vi "HIOKI PW3390 Acquisition Waveform.vi"() -> ()   [LabVIEW 2009]
doc: "Outputs the voltage and current waveforms of the specified channel."
uses:
  <instrlib>/PW3390/Common/_Initialize/HIOKI PW3390 Initialize LAN.vi
panel:
  out "error out":errorcluster
  in  "Analysis CH":enum16{"CH 1", "CH 2", "CH 3", "CH 4"}(ring)
  out "I Wave":waveform(sgl)(graph)
  out "U Wave":waveform(sgl)(graph)
  in  "IP Address":string="192.168.1.1"
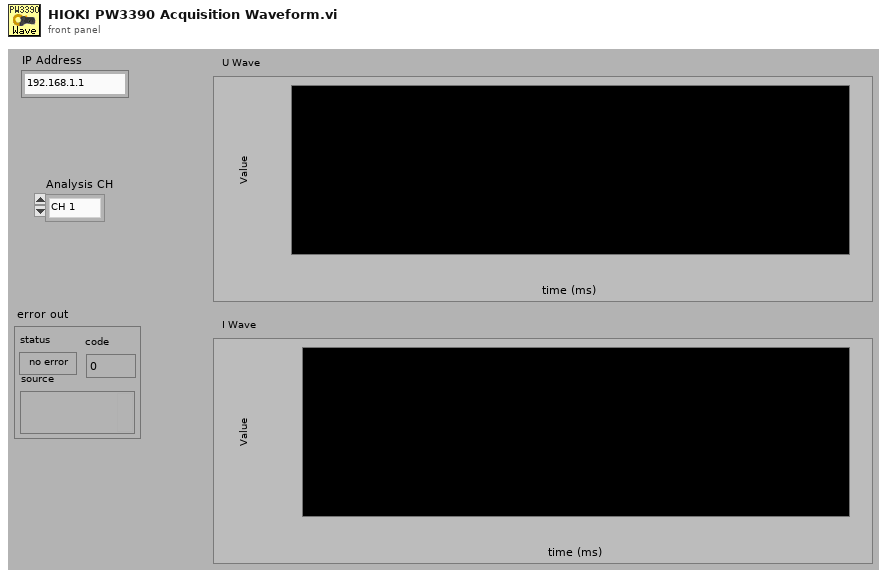
[diagram p1: front panel]
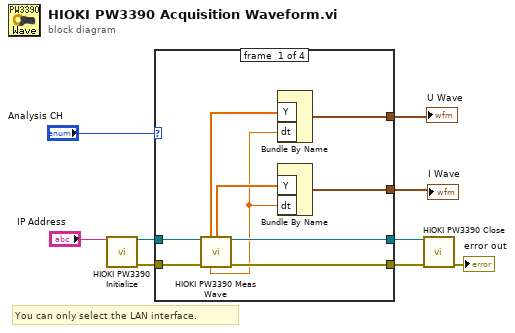
[diagram p0: block diagram]
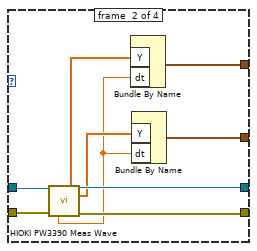
[diagram p2: hidden frame]
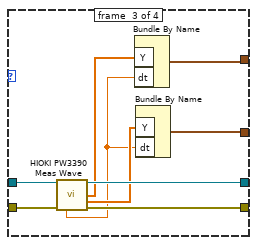
[diagram p3: hidden frame]
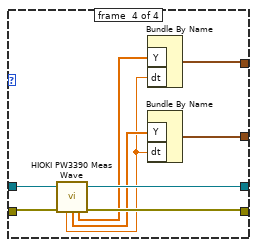
[diagram p4: hidden frame]
diagram:
  # "You can only select the LAN interface."
  n1 = call-poly <instrlib>:"HIOKI PW3390 Initialize.vi"("IP Address"="IP Address") -> ("VISA Resource out"=w5:refnum<visa-resource-name>, "error out"=w2:errorcluster)  [unwired: 12 in, 1 out]
  n2 = case shown="\"CH 1\"" "Analysis CH" {
    tunnel: [w18 w27 w36 w45] -> w7
    tunnel: [w17 w26 w35 w44] -> w6
    tunnel: w5 -> [w16 w25 w34 w43]
    tunnel: [w15 w22 w32 w40] -> w4
    tunnel: [w14 w23 w31 w41] -> w3
    tunnel: w2 -> [w13 w24 w33 w42]
    frame #0 {
      n3 = call <instrlib>:"HIOKI PW3390 Meas Wave.vi"("VISA Resource"=w16, "error in (no error)"=w13) -> ("U1 Value out"=w12:sgl[], "I1 Value out"=w11:sgl[], "VISA Resource out"=w15:refnum<visa-resource-name>, "dt out"=w10:dbl, "error out"=w14:errorcluster)  [unwired: 3 in, 6 out]
      n4 = Bundle By Name("Y"=w12, "dt"=w10) -> (w18:waveform(sgl))  [unwired: 1 in]
      n5 = Bundle By Name("Y"=w11, "dt"=w10) -> (w17:waveform(sgl))  [unwired: 1 in]
    }
    frame #1 {
      n6 = call <instrlib>:"HIOKI PW3390 Meas Wave.vi"("VISA Resource"=w25, "error in (no error)"=w24) -> ("U2 Value out"=w20:sgl[], "VISA Resource out"=w22:refnum<visa-resource-name>, "I2 Value out"=w21:sgl[], "dt out"=w19:dbl, "error out"=w23:errorcluster)  [unwired: 3 in, 6 out]
      n7 = Bundle By Name("Y"=w20, "dt"=w19) -> (w27:waveform(sgl))  [unwired: 1 in]
      n8 = Bundle By Name("Y"=w21, "dt"=w19) -> (w26:waveform(sgl))  [unwired: 1 in]
    }
    frame #2 {
      n9 = call <instrlib>:"HIOKI PW3390 Meas Wave.vi"("VISA Resource"=w34, "error in (no error)"=w33) -> ("VISA Resource out"=w32:refnum<visa-resource-name>, "U3 Value out"=w30:sgl[], "I3 Value out"=w29:sgl[], "dt out"=w28:dbl, "error out"=w31:errorcluster)  [unwired: 3 in, 6 out]
      n10 = Bundle By Name("Y"=w30, "dt"=w28) -> (w36:waveform(sgl))  [unwired: 1 in]
      n11 = Bundle By Name("Y"=w29, "dt"=w28) -> (w35:waveform(sgl))  [unwired: 1 in]
    }
    frame #3 {
      n12 = call <instrlib>:"HIOKI PW3390 Meas Wave.vi"("VISA Resource"=w43, "error in (no error)"=w42) -> ("VISA Resource out"=w40:refnum<visa-resource-name>, "dt out"=w37:dbl, "I4 Value out"=w38:sgl[], "U4 Value out"=w39:sgl[], "error out"=w41:errorcluster)  [unwired: 3 in, 6 out]
      n13 = Bundle By Name("Y"=w39, "dt"=w37) -> (w45:waveform(sgl))  [unwired: 1 in]
      n14 = Bundle By Name("Y"=w38, "dt"=w37) -> (w44:waveform(sgl))  [unwired: 1 in]
    }
  }
  "U Wave" <- w7
  "I Wave" <- w6
  n15 = call <instrlib>:"HIOKI PW3390 Close.vi"("VISA Resource"=w4, "error in (no error)"=w3) -> ("error out"=→"error out":errorcluster)  [unwired: 13 in]
